vi "Sys config window-Check valid setup.vi"() -> (1 "Continue":bool)   [LabVIEW 2020]
uses:
  Globals/Sys Config window globals.vi
  Typedefs/HW Setup tab control.ctl
  <userlib>/_OpenG.lib/array/array.llb/Remove Duplicates from 1D Array (String)__ogtk.vi
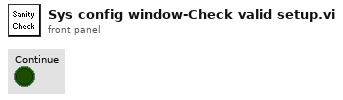
[diagram p1: front panel]
types:
  T1 = typedef "HW Setup tab control.ctl" = enum32{"Control System ", "DAQ FPGA", "Triggers", "HW Channels Setup", "XYZ stage", "Encoder", "Hardware Setup", "Cameras", "AOL Properties", "Calibration Settings", "Laser Settings", "PreChirper Settings", "General Setup"}
  T2 = typedef "HW config window refs cluster.ctl" = cluster{"VI's reference":refnum<vi>, "menu reference":refnum<k9>, "Pane":refnum<vi>, "Config Tab Control":refnum<vi>, "Triggers sub-tab control":refnum<vi>, "Microscope ID":refnum<vi>, "Microscope Type":refnum<vi>, "Revision Number":refnum<vi>, "Advanced Imaging":refnum<vi>, "Max Allowed Trial Length":refnum<vi>, "Initial Scan Resolution":refnum<vi>, "Initial Acceptance Angle":refnum<vi>, "Initial Laser Wavelength [nm] ":refnum<vi>, "Initial Dwell Time [us]":refnum<vi>, "Error Logging":refnum<vi>, "Performance Monitoring":refnum<vi>, "Ctrl FPGA available":refnum<vi>, "Control HW config":refnum<vi>, "Control System Config":refnum<vi>, "General trigger settings":refnum<vi>, "Trigger HW config":refnum<vi>, "Externalise Triggers":refnum<vi>, "[Triggers output setup]":refnum<vi>, "DAQ FPGA HW Config":refnum<vi>, "DAQ FPGA System Config":refnum<vi>, "Pockels AO":refnum<vi>, "Hard shutter AO":refnum<vi>, "PMT AOs":refnum<vi>, "Galvo AO":refnum<vi>, "Power meter AI":refnum<vi>, "PMT Voltage Lower Limit":refnum<vi>, "PMT Voltage Upper Limit":refnum<vi>, "XYZ Stage Control Config":refnum<vi>, "XY stage available":refnum<vi>, "XY Comms Config Cluster":refnum<vi>, "Y stage available":refnum<vi>, "Y Comms Config Cluster":refnum<vi>, "Z stage available":refnum<vi>, "Z Comms Config Cluster":refnum<vi>, "Encoder available":refnum<vi>, "Encoder":refnum<vi>, "Encoder IP address":refnum<vi>, "Encoder port":refnum<vi>, "Wheel radius (cm)":refnum<vi>, "Demo mode":refnum<vi>, "Swap XY on stage":refnum<vi>, "Number of AODs":refnum<vi>, "Axial MC Supported":refnum<vi>, "MC Supported":refnum<vi>, "Computer MAC add.":refnum<vi>, "Cam VidRec available":refnum<vi>, "Cam VidRec":refnum<vi>, "DO flag-Video record":refnum<vi>, "DO flag-Trial start":refnum<vi>, "AOD Settings (distilled)":refnum<vi>, "Pockels cal.Dwell time (µs)":refnum<vi>, "Pockels cal.Zoom":refnum<vi>, "Current Objective":refnum<vi>, "[Obj. Calib. Settings]":refnum<vi>, "Laser Wavelength":refnum<vi>, "Laser Power Control \nHW config":refnum<vi>, "Laser 1 available":refnum<vi>, "Laser 1 config":refnum<vi>, "Prechirper 1 available":refnum<vi>, "Prechirper 1 config":refnum<vi>, "PreChirp Preset Values":refnum<vi>, "[PreChirper Preset \nCalibration Values]":refnum<vi>, "Prechirper Constants":refnum<vi>}
  T3 = typedef "Control Sys HW config cluster.ctl" = cluster{"Control system.FPGA Type":enum16{"Virtex 5", "Virtex 7"}, "Control system.Network adapter name":string, "Control system.MAC address":string, "Control system.Ethernet Port":u32, "Control system.Ethernet Port Opened":bool}
  T4 = typedef "CTRL system config.ctl" = cluster{"AOD 1 Amplitude":i16, "AOD 2 Amplitude":i16, "AOD 3 Amplitude":i16, "AOD 4 Amplitude":i16, "AOD 5 Amplitude":i16, "AOD 6 Amplitude":i16, "T0 (ns)":dbl, "Ta (ns)":dbl, "Data Time Interval (ns)":dbl, "Ctrl FPGA Clock (MHz)":dbl}
  T5 = typedef "Triggers output setup.ctl" = T6[]
  T6 = typedef "Trigger setup element cluster.ctl" = cluster{"Name":string, "Output?":bool, "Output terminal":tag, "PXI backplane line":tag, "Pulse width (us)":u16}
  T7 = typedef "DAQ FPGA HW config cluster.ctl" = cluster{"FGPA Ref":T8, "Target":T9, "input card type":T10}
  T8 = typedef "FPGA Ref.ctl" = refnum<k20>
  T9 = typedef "nirio_resource_hc.ctl" = tag
  T10 = typedef "FPGA input type AC-DC.ctl" = enum16{"AC Card", "DC Card"}
  T11 = typedef "DAQ FPGA system config.ctl" = cluster{"Clock Freq (MHz) ":dbl, "Samples Wait after Trigger":u16, "AOD fill":u16, "StartupDelay":i32, "Slip Cycle (clock cycles)":u32, "Add Cycle":bool}
  T12 = typedef "Peripherals comms config cluster.ctl" = cluster{"Name":string, "Device Address":string, "Port ":u16, "Baudrate":i32, "Comms Type":T13}
  T13 = typedef "Comms Type.ctl" = enum16{"GPIB-IEEE488", "Serial-RS232", "Serial-RS485", "Serial-RS422", "Serial-USB", "Ethernet-TCP/IP", "Ethernet-UDP"}
  T14 = typedef "Encoder config cluster.ctl" = cluster{"IP address":string, "Port":u16, "Wheel radius (cm)":dbl, "Encoder Trigger":tag}
  T15 = typedef "Cam VidRec HW config setup cluster.ctl" = cluster{"DO flag-Video record":tag, "DO flag-Trial start":tag}
  T16 = typedef "Objective Config.ctl" = cluster{"Name":string, "Sum X":dbl, "Sum Y":dbl, "Diff X":dbl, "Diff Y":dbl, "Distortion Correction":dbl, "Z_norm to um_scaling":dbl, "X_norm to um_scaling":dbl, "Calibrated Wavelength":dbl}
  T17 = typedef "Laser 1 config cluster.ctl" = cluster{"COM port":refnum<visa-resource-name>, "Baud Rate":i32, "Type":string}
  T18 = typedef "PreChirper 1 config cluster.ctl" = cluster{"Type":string, "Baud Rate":i32, "COM port":refnum<visa-resource-name>}
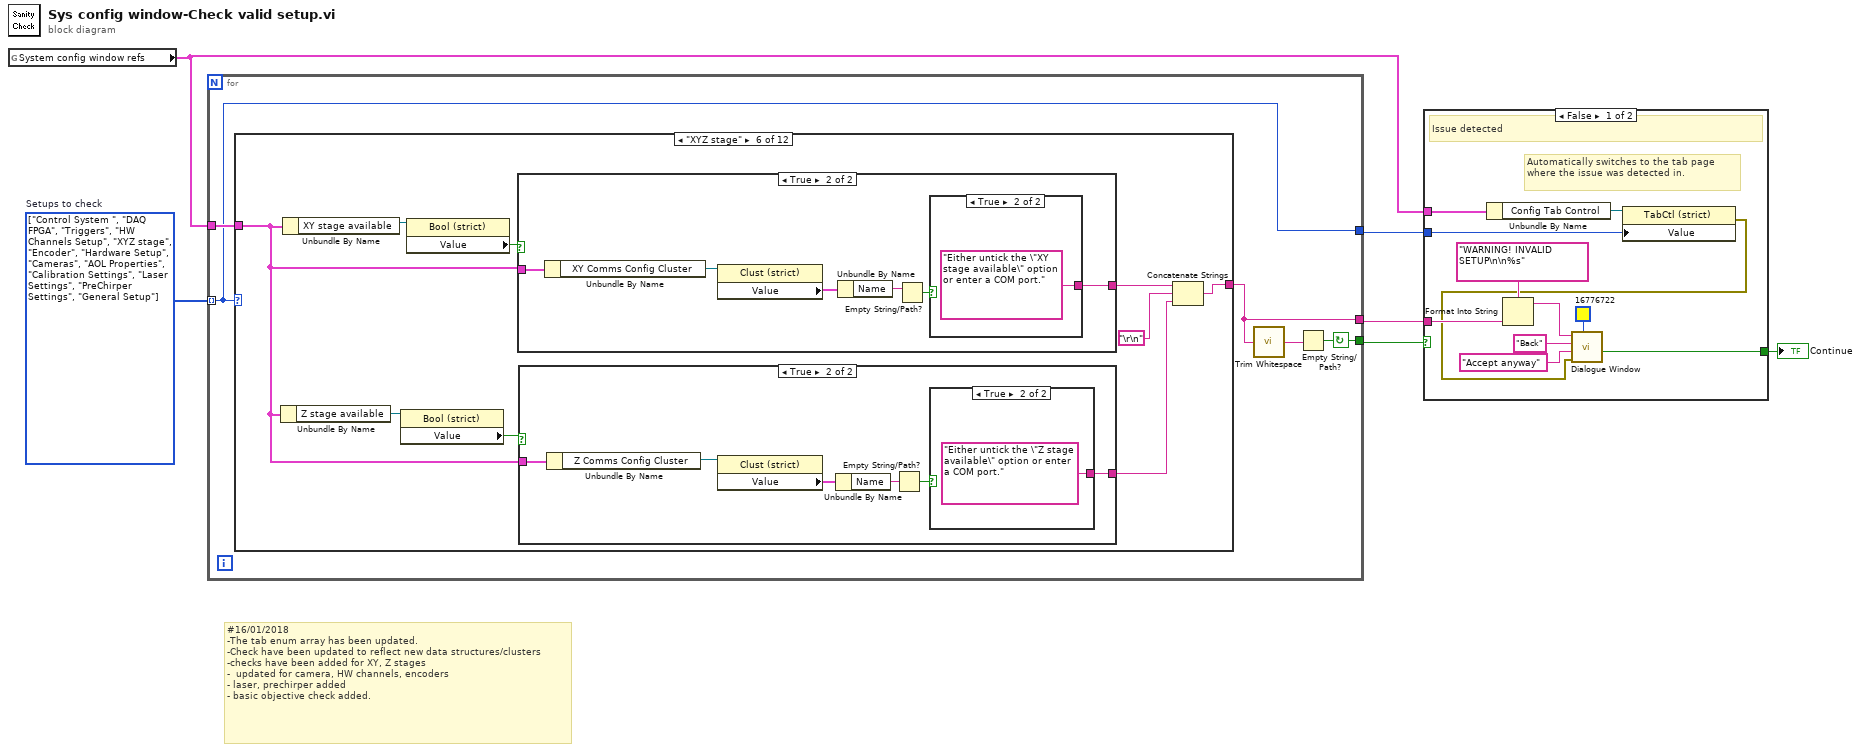
[diagram p0: block diagram]
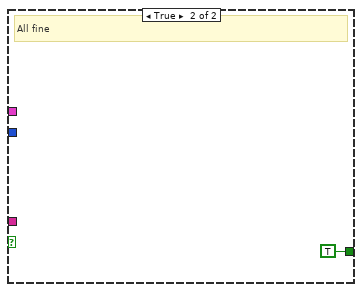
[diagram p2: hidden frame]
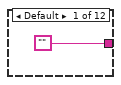
[diagram p3: hidden frame]
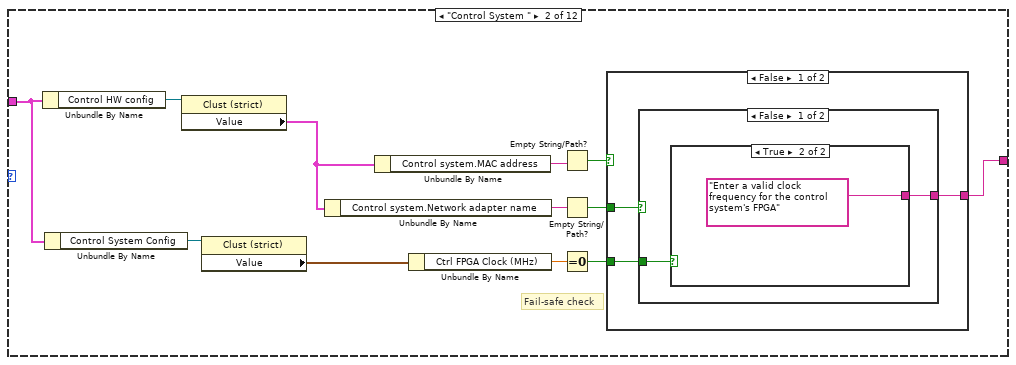
[diagram p4: hidden frame]
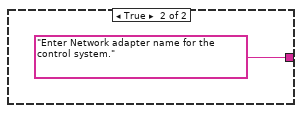
[diagram p6: hidden frame]
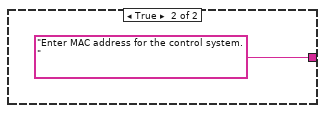
[diagram p7: hidden frame]
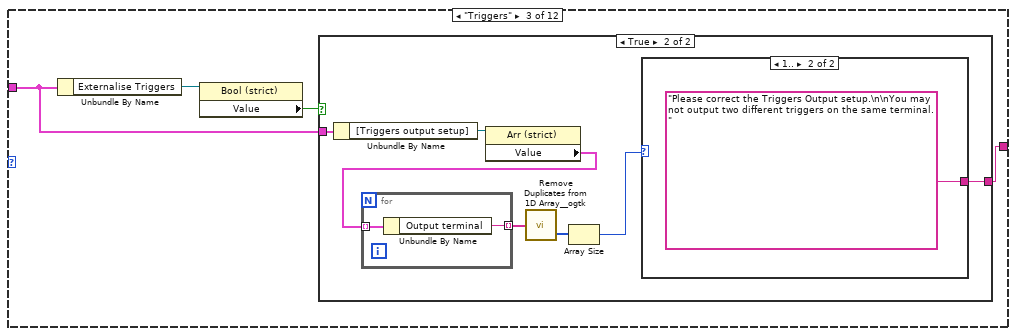
[diagram p8: hidden frame]
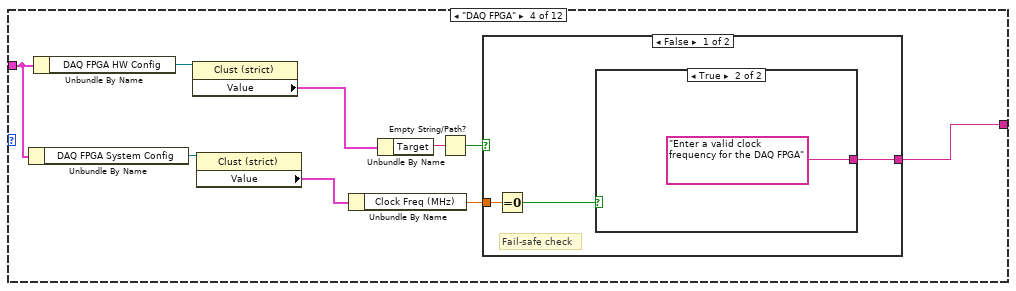
[diagram p11: hidden frame]
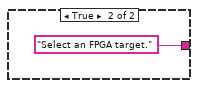
[diagram p13: hidden frame]
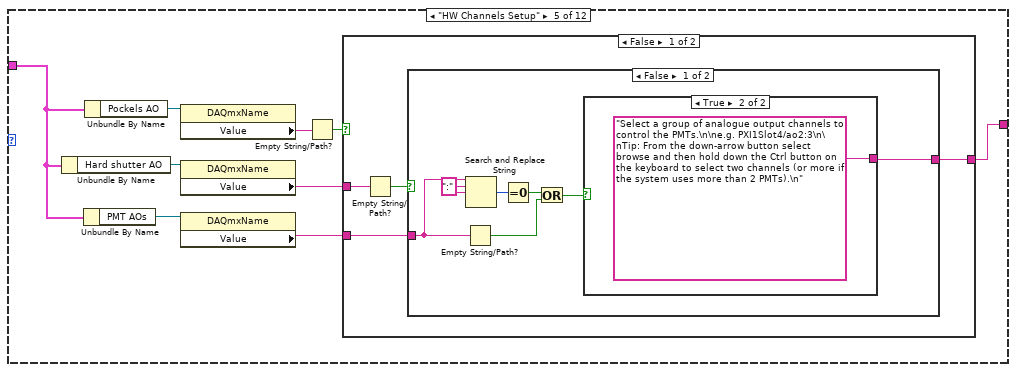
[diagram p14: hidden frame]
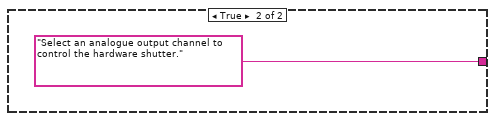
[diagram p16: hidden frame]
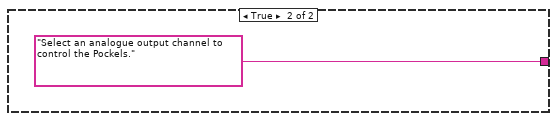
[diagram p17: hidden frame]
diagram:
  w1 = T1[] [enum."Control System ", enum."DAQ FPGA", enum."Triggers", enum."HW Channels Setup", enum."XYZ stage", enum."Encoder", enum."Hardware Setup", enum."Cameras", enum."AOL Properties", enum."Calibration Settings", enum."Laser Settings", enum."PreChirper Settings", enum."General Setup"] items=["Control System ", "DAQ FPGA", "Triggers", "HW Channels Setup", "XYZ stage", "Encoder", "Hardware Setup", "Cameras", "AOL Properties", "Calibration Settings", "Laser Settings", "PreChirper Settings", "General Setup"]  # Setups to check
  # "#16/01/2018\n-The tab enum array has been updated.\n-Check have been updated to reflect new data structures/clusters\n-checks have been added for XY, Z stages\n-  updated for camera, HW channels, encoders\n- laser, prechirper added\n- basic objective check added."
  n1 = global read "Sys Config window globals.vi" "System config window refs"() -> (w3:T2)
  n2 = for {
    tunnel: w3 -> [w11]
    tunnel: w1 -> [w9] mode=indexing
    tunnel: [w7] -> w5
    tunnel: [w9] -> w4
    tunnel: [w10] -> w6
    stop <- w10 continue-if-true
    n3 = case shown="\"XYZ stage\"" w9 {
      tunnel: w11 -> [_ w14 w36 w48 w62 w88 w110 w122 w127 w149 w155 w168]
      tunnel: ["" w24 w35 w55 w66 w84 w109 w121 w126 w138 w154 w167] -> w7
      frame Default {
      }
      frame "Control System " {
        # "Fail-safe check"
        n4 = Unbundle By Name(w14) -> ("Control HW config"=w20:refnum<vi>)
        n5 = Unbundle By Name(w14) -> ("Control System Config"=w15:refnum<vi>)
        n6 = property class="Clust (strict)"(reference=w20) -> ("Value"=w19:T3)  [unwired: 1 in, 2 out]
        n7 = property class="Clust (strict)"(reference=w15) -> ("Value"=w13:T4)  [unwired: 1 in, 2 out]
        n8 = Unbundle By Name(w19) -> ("Control system.Network adapter name"=w17:string)
        n9 = Unbundle By Name(w19) -> ("Control system.MAC address"=w18:string)
        n10 = Unbundle By Name(w13) -> ("Ctrl FPGA Clock (MHz)"=w16:dbl)
        n11 = Empty String/Path?(string/path=w18) -> (empty?=w23:bool)
        n12 = Empty String/Path?(string/path=w17) -> (empty?=w22:bool)
        n13 = Equal To 0?(x=w16) -> (x = 0?=w21:bool)
        n14 = case shown="False" w23 {
          tunnel: [w27 "Enter MAC address for the control system."] -> w24
          tunnel: w22 -> [w26 _]
          tunnel: w21 -> [w25 _]
          frame False {
            n15 = case shown="False" w26 {
              tunnel: [w29 "Enter Network adapter name for the control system."] -> w27
              tunnel: w25 -> [w28 _]
              frame False {
                n16 = case shown="True" w28 {
                  tunnel: [_ "Enter a valid clock frequency for the control system's FPGA"] -> w29
                  frame False {
                  }
                  frame True {
                  }
                }
              }
              frame True {
              }
            }
          }
          frame True {
          }
        }
      }
      frame "Triggers" {
        n17 = Unbundle By Name(w36) -> ("Externalise Triggers"=w34:refnum<vi>)
        n18 = property class="Bool (strict)"(reference=w34) -> ("Value"=w33:bool)  [unwired: 1 in, 2 out]
        n19 = case shown="True" w33 {
          tunnel: w36 -> [_ w42]
          tunnel: [_ w41] -> w35
          frame False {
          }
          frame True {
            n20 = Unbundle By Name(w42) -> ("[Triggers output setup]"=w43:refnum<vi>)
            n21 = property class="Arr (strict)"(reference=w43) -> ("Value"=w40:T5)  [unwired: 1 in, 2 out]
            n22 = for {
              tunnel: w40 -> [w45] mode=indexing
              tunnel: [w44] -> w39 mode=indexing
              n23 = Unbundle By Name(w45) -> ("Output terminal"=w44:tag)
            }
            n24 = call-poly <userlib>:"Remove Duplicates from 1D Array__ogtk.vi"("Input Array"=w39) -> ("indices of removed elements"=w38:i32[])  [unwired: 1 out]
            n25 = Array Size(array=w38) -> (size(s)=w37:i32)
            n26 = case shown="1.." w37 {
              tunnel: [_ "Please correct the Triggers Output setup.\n\nYou may not output two different triggers on the same terminal."] -> w41
              frame 0, Default {
              }
              frame 1.. {
              }
            }
          }
        }
      }
      frame "DAQ FPGA" {
        n27 = Unbundle By Name(w48) -> ("DAQ FPGA System Config"=w49:refnum<vi>)
        n28 = Unbundle By Name(w48) -> ("DAQ FPGA HW Config"=w53:refnum<vi>)
        n29 = property class="Clust (strict)"(reference=w53) -> ("Value"=w52:T7)  [unwired: 1 in, 2 out]
        n30 = property class="Clust (strict)"(reference=w49) -> ("Value"=w47:T11)  [unwired: 1 in, 2 out]
        n31 = Unbundle By Name(w47) -> ("Clock Freq (MHz)"=w50:dbl)
        n32 = Unbundle By Name(w52) -> ("Target"=w51:T9)
        n33 = Empty String/Path?(string/path=w51) -> (empty?=w54:bool)
        n34 = case shown="False" w54 {
          tunnel: [w56 "Select an FPGA target."] -> w55
          tunnel: w50 -> [w58 _]
          frame False {
            # "Fail-safe check"
            n35 = Equal To 0?(x=w58) -> (x = 0?=w57:bool)
            n36 = case shown="True" w57 {
              tunnel: [_ "Enter a valid clock frequency for the DAQ FPGA"] -> w56
              frame False {
              }
              frame True {
              }
            }
          }
          frame True {
          }
        }
      }
      frame "HW Channels Setup" {
        n37 = Unbundle By Name(w62) -> ("Hard shutter AO"=w69:refnum<vi>)
        n38 = Unbundle By Name(w62) -> ("PMT AOs"=w63:refnum<vi>)
        n39 = Unbundle By Name(w62) -> ("Pockels AO"=w68:refnum<vi>)
        n40 = property class="DAQmxName"(reference=w68) -> ("Value"=w67:string)  [unwired: 1 in, 2 out]
        n41 = property class="DAQmxName"(reference=w69) -> ("Value"=w64:string)  [unwired: 1 in, 2 out]
        n42 = property class="DAQmxName"(reference=w63) -> ("Value"=w61:string)  [unwired: 1 in, 2 out]
        n43 = Empty String/Path?(string/path=w67) -> (empty?=w65:bool)
        n44 = case shown="False" w65 {
          tunnel: [w73 "Select an analogue output channel to control the Pockels."] -> w66
          tunnel: w64 -> [w72 _]
          tunnel: w61 -> [w70 _]
          frame False {
            n45 = Empty String/Path?(string/path=w72) -> (empty?=w71:bool)
            n46 = case shown="False" w71 {
              tunnel: [w80 "Select an analogue output channel to control the hardware shutter."] -> w73
              tunnel: w70 -> [w79 _]
              frame False {
                w78 = ":" ("search string")
                n47 = Empty String/Path?(string/path=w79) -> (empty?=w75:bool)
                n48 = Search and Replace String(input string=w79, search string=w78, replace string=w78) -> (number of replacements=w77:i32)  [unwired: 5 in, 3 out]
                n49 = Equal To 0?(x=w77) -> (x = 0?=w76:bool)
                n50 = Or(x=w76, y=w75) -> (x .or. y?=w74:bool)
                n51 = case shown="True" w74 {
                  tunnel: [_ "Select a group of analogue output channels to control the PMTs.\n\ne.g. PXI1Slot4/ao2:3\n\nTip: From the down-arrow button select browse and then hold down the Ctrl button on the keyboard to select two channels (or more if the system uses more than 2 PMTs).\n"] -> w80
                  frame False {
                  }
                  frame True {
                  }
                }
              }
              frame True {
              }
            }
          }
          frame True {
          }
        }
      }
      frame "XYZ stage" {
        n52 = Unbundle By Name(w88) -> ("Z stage available"=w89:refnum<vi>)
        n53 = Unbundle By Name(w88) -> ("XY stage available"=w92:refnum<vi>)
        n54 = property class="Bool (strict)"(reference=w89) -> ("Value"=w90:bool)  [unwired: 1 in, 2 out]
        n55 = property class="Bool (strict)"(reference=w92) -> ("Value"=w91:bool)  [unwired: 1 in, 2 out]
        n56 = case shown="True" w91 {
          tunnel: w88 -> [_ w104]
          tunnel: [_ w103] -> w87
          frame False {
          }
          frame True {
            n57 = Unbundle By Name(w104) -> ("XY Comms Config Cluster"=w105:refnum<vi>)
            n58 = property class="Clust (strict)"(reference=w105) -> ("Value"=w101:T12)  [unwired: 1 in, 2 out]
            n59 = Unbundle By Name(w101) -> ("Name"=w100:string)
            n60 = Empty String/Path?(string/path=w100) -> (empty?=w102:bool)
            n61 = case shown="True" w102 {
              tunnel: [_ "Either untick the \"XY stage available\" option or enter a COM port."] -> w103
              frame False {
              }
              frame True {
              }
            }
          }
        }
        n62 = case shown="True" w90 {
          tunnel: w88 -> [_ w97]
          tunnel: [_ w96] -> w85
          frame False {
          }
          frame True {
            n63 = Unbundle By Name(w97) -> ("Z Comms Config Cluster"=w98:refnum<vi>)
            n64 = property class="Clust (strict)"(reference=w98) -> ("Value"=w95:T12)  [unwired: 1 in, 2 out]
            n65 = Unbundle By Name(w95) -> ("Name"=w94:string)
            n66 = Empty String/Path?(string/path=w94) -> (empty?=w93:bool)
            n67 = case shown="True" w93 {
              tunnel: [_ "Either untick the \"Z stage available\" option or enter a COM port."] -> w96
              frame False {
              }
              frame True {
              }
            }
          }
        }
        n68 = Concatenate Strings(w87, "\r\n", w85) -> (w84:string)
      }
      frame "Encoder" {
        n69 = Unbundle By Name(w110) -> ("Encoder available"=w108:refnum<vi>)
        n70 = property class="Bool (strict)"(reference=w108) -> ("Value"=w107:bool)  [unwired: 1 in, 2 out]
        n71 = case shown="True" w107 {
          tunnel: w110 -> [_ w115]
          tunnel: [_ w114] -> w109
          frame False {
          }
          frame True {
            n72 = Unbundle By Name(w115) -> ("Encoder"=w116:refnum<vi>)
            n73 = property class="Clust (strict)"(reference=w116) -> ("Value"=w112:T14)  [unwired: 1 in, 2 out]
            n74 = Unbundle By Name(w112) -> ("IP address"=w111:string)
            n75 = Empty String/Path?(string/path=w111) -> (empty?=w113:bool)
            n76 = case shown="True" w113 {
              tunnel: [_ "Either untick the \"Encoder available\" option or enter the encoder's IP address."] -> w114
              frame False {
              }
              frame True {
              }
            }
          }
        }
      }
      frame "Hardware Setup" {
        n77 = Unbundle By Name(w122) -> ("Computer MAC add."=w120:refnum<vi>)
        n78 = property class="Str"(reference=w120) -> ("Value"=w119:string)  [unwired: 1 in, 2 out]
        n79 = Empty String/Path?(string/path=w119) -> (empty?=w118:bool)
        n80 = case shown="True" w118 {
          tunnel: [_ "Enter this computer's MAC address.\nThis is required to establish connection with the control system."] -> w121
          frame False {
          }
          frame True {
          }
        }
      }
      frame "Cameras" {
        n81 = Unbundle By Name(w127) -> ("Cam VidRec available"=w125:refnum<vi>)
        n82 = property class="Bool (strict)"(reference=w125) -> ("Value"=w124:bool)  [unwired: 1 in, 2 out]
        n83 = case shown="True" w124 {
          tunnel: w127 -> [_ w135]
          tunnel: [_ w131] -> w126
          frame False {
          }
          frame True {
            n84 = Unbundle By Name(w135) -> ("Cam VidRec"=w136:refnum<vi>)
            n85 = property class="Clust (strict)"(reference=w136) -> ("Value"=w130:T15)  [unwired: 1 in, 2 out]
            n86 = Unbundle By Name(w130) -> ("DO flag-Video record"=w129:tag, "DO flag-Trial start"=w128:tag)
            n87 = Empty String/Path?(string/path=w129) -> (empty?=w133:bool)
            n88 = Empty String/Path?(string/path=w128) -> (empty?=w134:bool)
            n89 = Compound Arithmetic op=OR(w133, w134) -> (w132:bool)
            n90 = case shown="True" w132 {
              tunnel: [_ "Either untick the\n\"Cameras video recording system is available\" option or specify valid digital output channels."] -> w131
              frame False {
              }
              frame True {
              }
            }
          }
        }
      }
      frame "Calibration Settings" {
        n91 = Unbundle By Name(w149) -> ("Current Objective"=w148:refnum<vi>, "[Obj. Calib. Settings]"=w147:refnum<vi>)
        n92 = property class="Arr (strict)"(reference=w147) -> ("Value"=w146:T16[])  [unwired: 1 in, 2 out]
        n93 = for {
          tunnel: w146 -> [w151] mode=indexing
          tunnel: [w150] -> w145 mode=indexing
          n94 = Unbundle By Name(w151) -> ("Name"=w150:string)
        }
        n95 = property class="Str"(reference=w148) -> ("Value"=w144:string)  [unwired: 1 in, 2 out]
        n96 = Empty String/Path?(string/path=w144) -> (empty?=w141:bool)
        n97 = Search 1D Array(1D array=w145, element=w144) -> (index of element=w143:i32)  [unwired: 1 in]
        n98 = Equal?(x=w143, y=-1) -> (x = y?=w140:bool)
        n99 = Or(x=w141, y=w140) -> (x .or. y?=w139:bool)
        n100 = case shown="False" w139 {
          tunnel: ["" "Correct Objective not selected OR settings not found for the objective.\nPlease change and reload the calibration file."] -> w138
          frame False {
          }
          frame True {
          }
        }
      }
      frame "Laser Settings" {
        n101 = Unbundle By Name(w155) -> ("Laser 1 available"=w157:refnum<vi>)
        n102 = property class="Bool (strict)"(reference=w157) -> ("Value"=w156:bool)  [unwired: 1 in, 2 out]
        n103 = case shown="True" w156 {
          tunnel: w155 -> [_ w163]
          tunnel: ["" w162] -> w154
          frame False {
          }
          frame True {
            n104 = Unbundle By Name(w163) -> ("Laser 1 config"=w164:refnum<vi>)
            n105 = property class="Clust (strict)"(reference=w164) -> ("Value"=w160:T17)  [unwired: 1 in, 2 out]
            n106 = Unbundle By Name(w160) -> ("COM port"=w159:refnum<visa-resource-name>)
            n107 = Empty String/Path?(string/path=w159) -> (empty?=w161:bool)
            n108 = case shown="False" w161 {
              tunnel: ["" "Either untick the \"Laser 1 available\" option or enter a COM port."] -> w162
              frame False {
              }
              frame True {
              }
            }
          }
        }
      }
      frame "PreChirper Settings" {
        n109 = Unbundle By Name(w168) -> ("Prechirper 1 available"=w170:refnum<vi>)
        n110 = property class="Bool (strict)"(reference=w170) -> ("Value"=w169:bool)  [unwired: 1 in, 2 out]
        n111 = case shown="True" w169 {
          tunnel: w168 -> [_ w176]
          tunnel: ["" w175] -> w167
          frame False {
          }
          frame True {
            n112 = Unbundle By Name(w176) -> ("Prechirper 1 config"=w177:refnum<vi>)
            n113 = property class="Clust (strict)"(reference=w177) -> ("Value"=w173:T18)  [unwired: 1 in, 2 out]
            n114 = Unbundle By Name(w173) -> ("COM port"=w172:refnum<visa-resource-name>)
            n115 = Empty String/Path?(string/path=w172) -> (empty?=w174:bool)
            n116 = case shown="False" w174 {
              tunnel: ["" "Either untick the \"Laser 1 available\" option or enter a COM port."] -> w175
              frame False {
              }
              frame True {
              }
            }
          }
        }
      }
    }
    n117 = call <vilib>:"Trim Whitespace.vi"("string"=w7) -> ("trimmed string"=w8:string)  [unwired: 1 in]
    n118 = Empty String/Path?(string/path=w8) -> (empty?=w10:bool)
  }
  n119 = case shown="False" w6 {
    tunnel: w5 -> [w187 _]
    tunnel: w4 -> [w180 _]
    tunnel: w3 -> [w190 _]
    tunnel: [w183 TRUE] -> w2
    frame False {
      # "Automatically switches to the tab page where the issue was detected in."
      # "Issue detected"
      n120 = Unbundle By Name(w190) -> ("Config Tab Control"=w189:refnum<vi>)
      n121 = Format Into String(format string="WARNING! INVALID SETUP\n\n%s" ("Message string"), w187) -> (resulting string=w186:string)  [unwired: 2 in, 1 out]
      n122 = property class="TabCtl (strict)"(reference=w189, "Value"=w180) -> (error out=w181:errorcluster)  [unwired: 1 in, 1 out]
      n123 = call "Dialogue Window.vi"("Colour"=u32 16776722, "error in (no error)"=w181, "Caption-Left button (Cancel)"="Accept anyway", "Caption-Right button (OK)"="Back", "Message string"=w186) -> ("Cancelled (Left button pressed)"=w183:bool)  [unwired: 4 in, 2 out]
    }
    frame True {
      # "All fine"
    }
  }
  "Continue" <- w2
